vi "Define Test Suite (SimpleText Report).vi"(4 "timeout":i32=2000, 6 "Verbose (F)":bool, 8 "error in (no error)":errorcluster, 9 "Report Path":path, 10 "Interactive":bool, 11 "Label (VI Title)":string) -> (0 "error out":errorcluster, 2 "Properties.Suite":refnum<class "Properties.Suite.lvclass">, 3 "Test Suite":refnum<class "Test Suite.lvclass">)   [LabVIEW 2013, in "Caraya.lvlib" / "Test Suite.lvclass"]
doc: "Registers the calling VI as a test suite. If Interactive is True, the interactive user interface is opened when the test suite is executed. If the Report Path is set, a report file will be generated with the test results.\n\n--\nCopyright © 2015 JKI All rights reserved.\n\nAuthor: Tomi Maila <tomi.maila@jki.net>\n\nThis library is provided \"AS IS\" ,WITHOUT WARRANTIES OR\nCONDITIONS OF ANY KIND, either express or implied.\n\nJKI -- jki.net"
uses:
  Test Suite.lvclass
  Properties.Suite/Properties.Suite.lvclass
  Test Assert Factory/Test Assert Factory.lvclass
  Test Report.Default/Test Report.Default.lvclass
  Test Suite.lvclass/Test Suite.ctl
  Properties.Suite/Properties.Suite.lvclass/Properties.Suite.ctl
  Caraya.lvlib
  Assert Factory Manager/Assert Factory Manager.lvclass
  Basic Test Manager/Basic Test Manager.lvclass
  Properties/Properties.lvclass
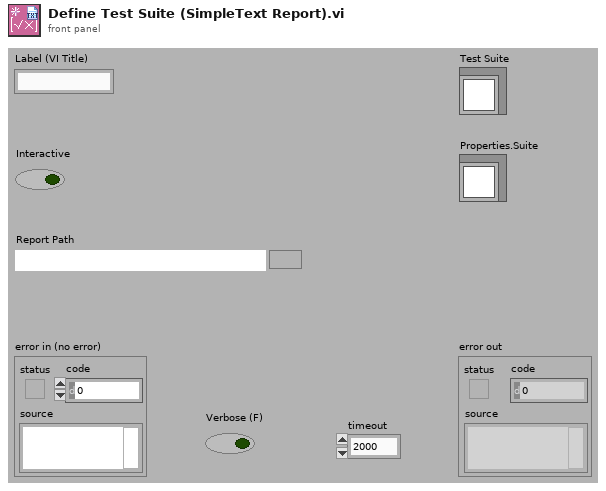
[diagram p1: front panel]
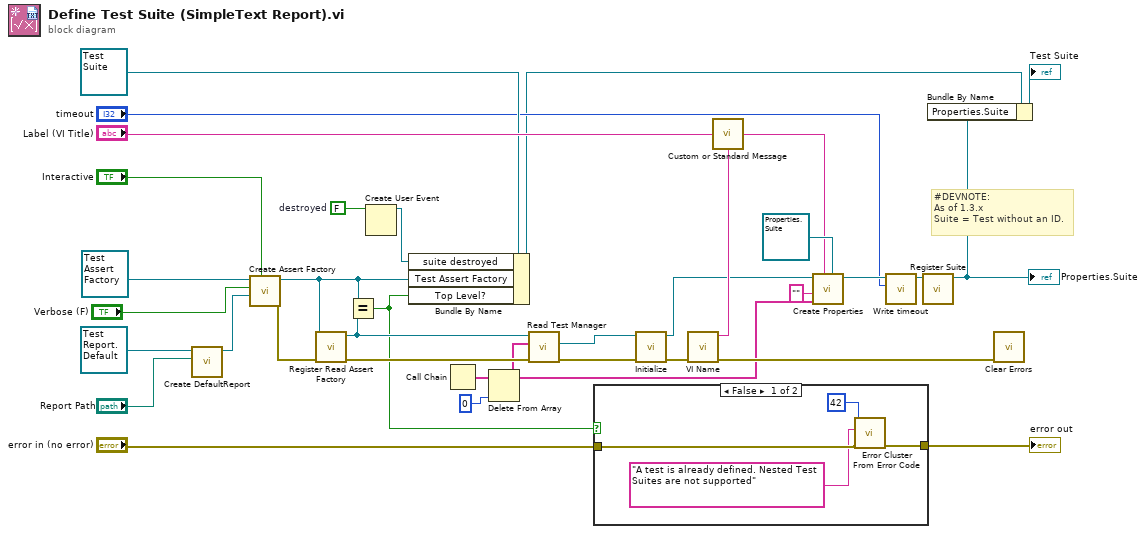
[diagram p0: block diagram]
diagram:
  w13 = FALSE  # destroyed
  # "#DEVNOTE:\nAs of 1.3.x\nSuite = Test without an ID."
  n1 = call "Create DefaultReport.vi"("Report Path"="Report Path", "Test Report.Default in"=refnum<class "Test Report.Default.lvclass"> refnum) -> ("Test Report.Default out"=w17:refnum<class "Test Report.Default.lvclass">)  [unwired: 8 in, 1 out]
  n2 = call "Create Assert Factory.vi"("Interactive"="Interactive", "Test Report"=w17, "Verbose (F)"="Verbose (F)", "Test Assert Factory in"=refnum<class "Test Assert Factory.lvclass"> refnum ("Caraya.lvlib:Test Assert Factory.lvclass")) -> ("error out"=w15:errorcluster, "Test Assert Factory out"=w16:refnum<class "Test Assert Factory.lvclass">)  [unwired: 6 in]
  n3 = call "Register Read Assert Factory.vi"("error in (no error)"=w15, "Test Assert Factory"=w16) -> ("error out"=w34:errorcluster, "Test Assert Factory"=w27:refnum<class "Test Assert Factory.lvclass">)  [unwired: 8 in]
  n4 = Equal?(x=w16, y=w27) -> (x = y?=w14:bool)
  n5 = Create User Event(user event datatype=w13) -> (user event=w12:refnum<user-event>)  [unwired: 1 in, 1 out]
  n6 = Bundle By Name(cluster=refnum<class "Test Suite.lvclass"> refnum ("Test Suite"), "suite destroyed"=w12, "Test Assert Factory"=w16, "Top Level?"=w14) -> (w2:refnum<class "Test Suite.lvclass">)
  n7 = Call Chain() -> (call chain=w28:string[])
  n8 = Delete From Array(array=w28, index=0) -> (array with subset deleted=w8:string[])  [unwired: 1 in, 1 out]
  n9 = call-dynamic "Read Test Manager.vi"("error in (no error)"=w34, "VI Call Chain"=w8, "Assert Factory in"=w27) -> ("error out"=w32:errorcluster, "Basic Test Manager"=w24:refnum<class "Basic Test Manager.lvclass">)  [unwired: 6 in, 1 out]
  n10 = case shown="False" w14 {
    tunnel: [w39 w40] -> w26
    tunnel: "error in (no error)" -> [w38 w40]
    frame False {
      n11 = call <vilib>:"Error Cluster From Error Code.vi"("error in (no error)"=w38, "error message (\"\")"="A test is already defined. Nested Test Suites are not supported" ("error message (\"\")"), "error code (0)"=42) -> ("error out"=w39:errorcluster)  [unwired: 6 in]
    }
    frame True {
    }
  }
  "error out" <- w26
  n12 = call "Initialize.vi"("error in (no error)"=w32, "Test Manager in"=w24) -> ("error out"=w31:errorcluster, "Test Manager out"=w7:refnum<class "Basic Test Manager.lvclass">)  [unwired: 8 in]
  n13 = call "VI Name.vi"("error in (no error)"=w31) -> ("error out"=w30:errorcluster, "VI Name"=w33:string)  [unwired: 9 in]
  n14 = call "Custom or Standard Message.vi"("Custom Message"="Label (VI Title)", "Standard Message"=w33) -> ("Message"=w9:string)
  n15 = call "Create Properties.vi"("Properties in"=refnum<class "Properties.Suite.lvclass"> refnum ("Caraya.lvlib:Properties.Suite.lvclass"), "label"=w9, "call-chain"=w8, "self-id"="", "Test Manager"=w7) -> ("Properties out"=w6:refnum<class "Properties.Suite.lvclass">)  [unwired: 6 in]
  n16 = call "Write timeout.vi"("timeout"="timeout", "Properties.Suite in"=w6) -> ("Properties.Suite out"=w5:refnum<class "Properties.Suite.lvclass">)  [unwired: 9 in]
  n17 = call "Register Suite.vi"("Properties.Suite in"=w5) -> ("Properties.Suite out"=w3:refnum<class "Properties.Suite.lvclass">)  [unwired: 10 in]
  "Properties.Suite" <- w3
  n18 = Bundle By Name(cluster=w2, "Properties.Suite"=w3) -> (→"Test Suite":refnum<class "Test Suite.lvclass">)
  n19 = call <vilib>:"Clear Errors.vi"("error in (no error)"=w30) -> ()  [unwired: 6 in, 1 out]
